vi "ECC.vi"() -> ()   [LabVIEW 2013]
uses:
  state_machine.ctl
  <vilib>/DAQmx/write.llb/DAQmx Write (Analog Wfm 1Chan NSamp).vi
  <vilib>/DAQmx/create/channels.llb/DAQmx Create Channel (AO-Voltage-Basic).vi
  <vilib>/DAQmx/configure/timing.llb/DAQmx Timing (Use Waveform).vi
  <vilib>/DAQmx/miscellaneous.llb/DAQmx Fill In Error Info.vi
panel:
  out "on_bad_status":bool
  out "off_bad_status":bool
  out "Pause, s":i32
  out "APS_off_status":bool=TRUE
  out "R&S_off_status":bool=TRUE
  out "Countdown":u32
  in  "Rep_delay":u32
  in  "Finite/Continuous":bool
  in  "ResumeSweep":bool
  in  "PauseSweep":bool
  in  "R&S_off_rep":bool
  in  "R&S_off_set":bool
  in  "R&S_off_cycle":bool
  in  "APS_off_rep":bool=TRUE
  in  "APS_off_set":bool
  in  "APS_off_cycle":bool
  in  "AbortSweep":bool
  in  "Check APS":bool
  in  "ON/OFF_APS":bool
  in  "Check R&S":bool
  in  "ON/OFF_R&S":bool
  in  "Use_APS":bool=TRUE
  out "DAC_status":bool
  out "R&S_status":bool
  out "i_Current_repetition":i32
  out "N_Cycles_Created":i32
  out "i_Current_cycle":i32
  in  "M_repetitions":i32 min=0
  in  "Set_of_Cycles":T1(array[cluster])=[{"On/Off"=TRUE, "f0, MHz"=32.5, "fm, kHz"=100.0, "A, mV"=20.0, "Waveform"=enum."triangle", "N_steps"=500, "T_sweep, s"=0.1, "N_sweeps"=5, "End_Wait, s"=0}] {"End_Wait, s" step=1; "N_sweeps" min=0 step=1; "T_sweep, s" min=0.0 step=0.001 format="%#_6f"; "N_steps" min=0 step=1; "fm, kHz" step=1.0; "f0, MHz" min=0.0 step=0.001 format="%#_6f"}
  out "APS_status":bool
  in  "APS address":refnum<visa-resource-name>="COM3"
  in  "Init Devices":bool
  in  "Do Sweep":bool
  in  "Exit":bool
  in  "DAC channel":tag="Dev1/ao0"
  in  "R&S address":string="29"
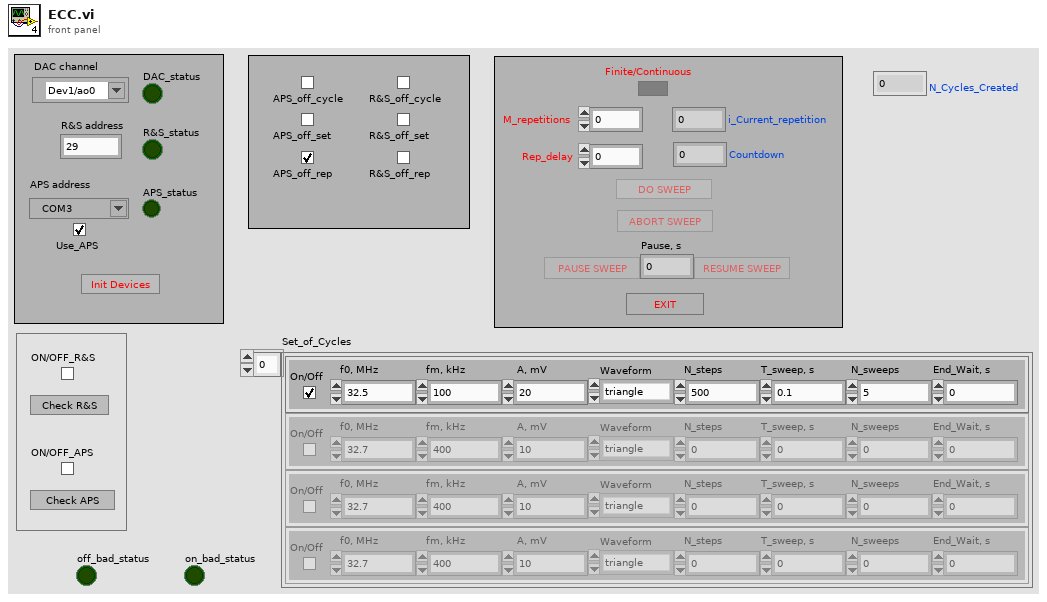
[diagram p1: front panel]
types:
  T1 = cluster{"On/Off":bool, "f0, MHz":dbl, "fm, kHz":dbl, "A, mV":dbl, "Waveform":enum16{"triangle", "saw_direct", "saw_invert", "sine"}, "N_steps":i32, "T_sweep, s":dbl, "N_sweeps":i32, "End_Wait, s":u32}[]
  T2 = typedef "state_machine.ctl" = enum16{"idle", "init_daq", "init_rf", "init_ps", "cycle_start", "get_wf", "rf_on", "rf_off", "rf_set", "ps_on", "ps_off", "daq_start", "daq_stop", "daq_wait", "daq_dt", "daq_v", "delay", "cycle_reset", "exit", "repetition_reset"}
  T3 = enum8{"Enabled", "Disabled", "Disabled and Grayed Out"}
  T4 = cluster{"On/Off":bool, "f0, MHz":dbl, "fm, kHz":dbl, "A, mV":dbl, "Waveform":enum16{"triangle", "saw_direct", "saw_invert", "sine"}, "N_steps":i32, "T_sweep, s":dbl, "N_sweeps":i32, "End_Wait, s":u32}
  T5 = enum16{"triangle", "saw_direct", "saw_invert", "sine"}
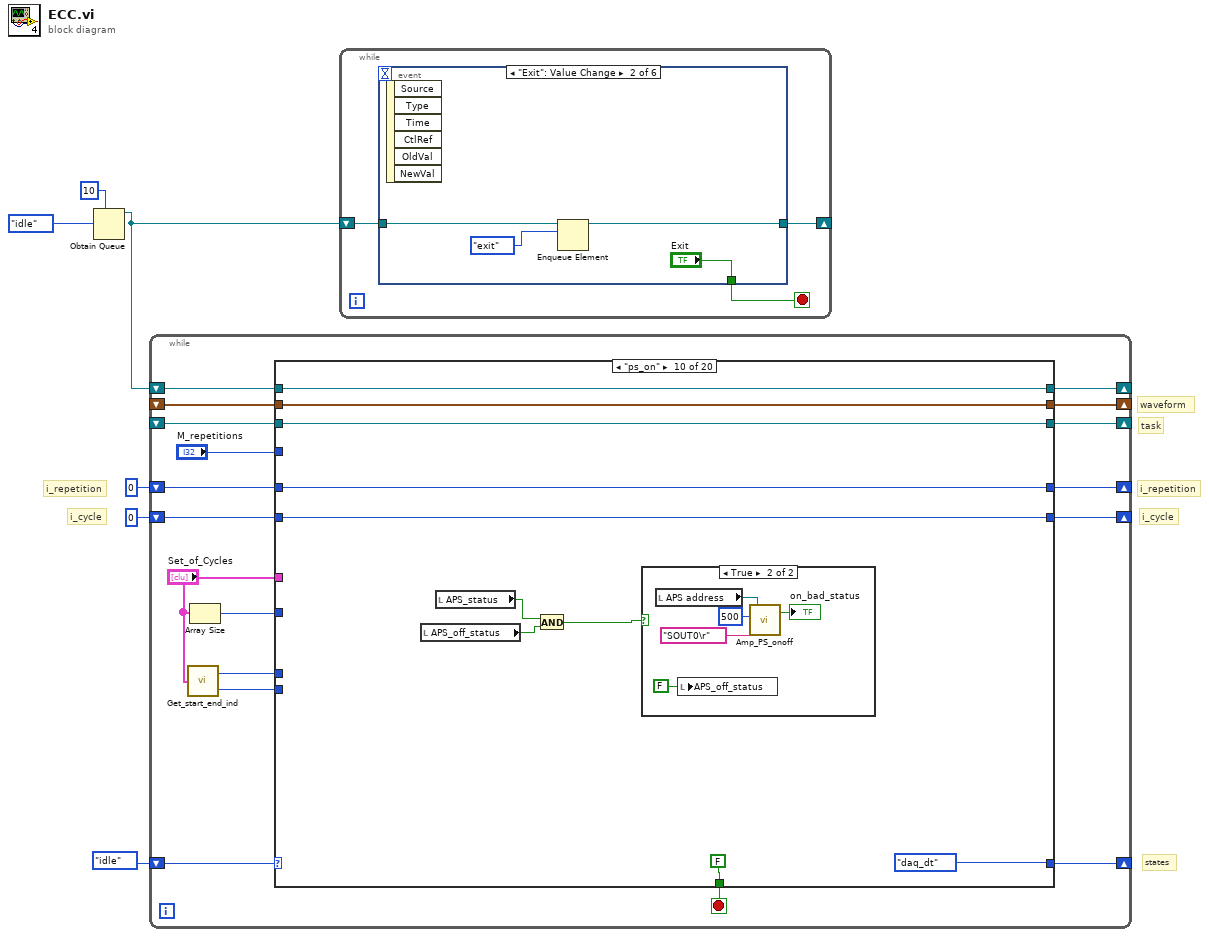
[diagram p0: block diagram]
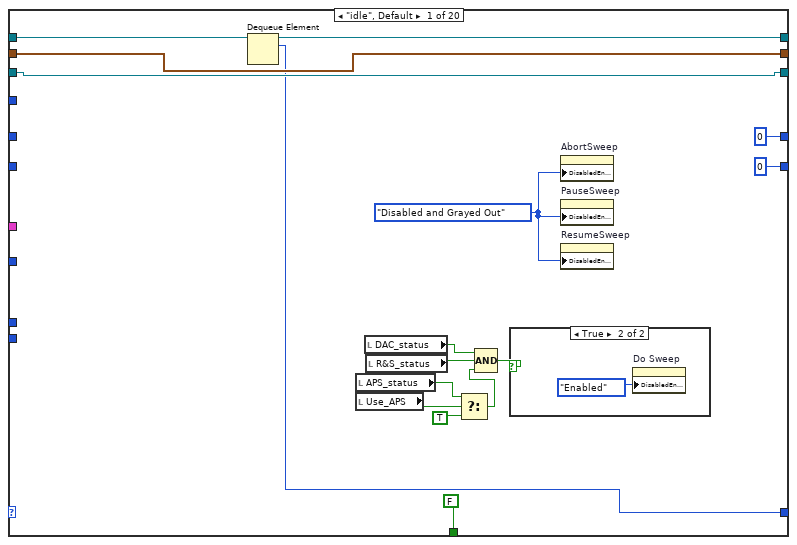
[diagram p2: hidden frame]
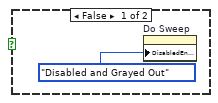
[diagram p3: hidden frame]
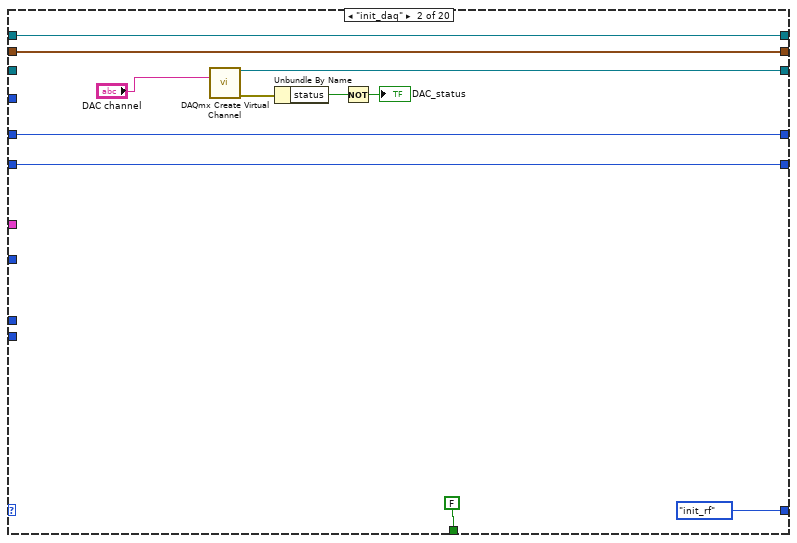
[diagram p4: hidden frame]
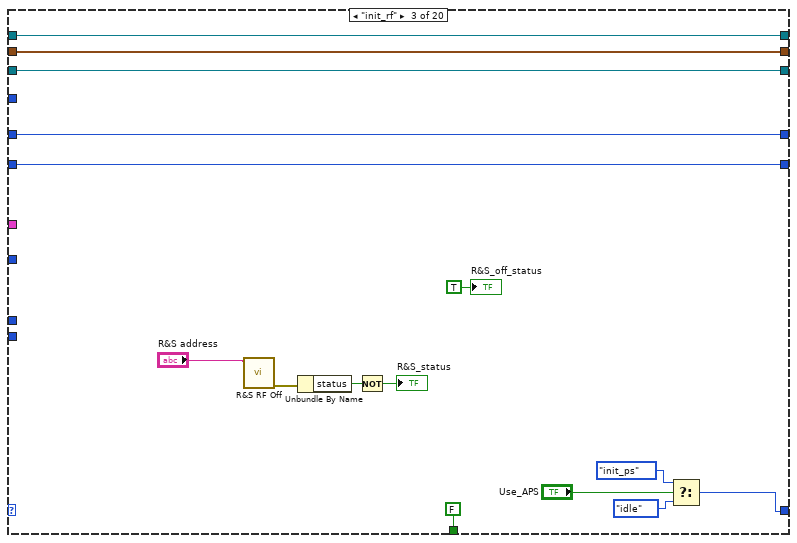
[diagram p5: hidden frame]
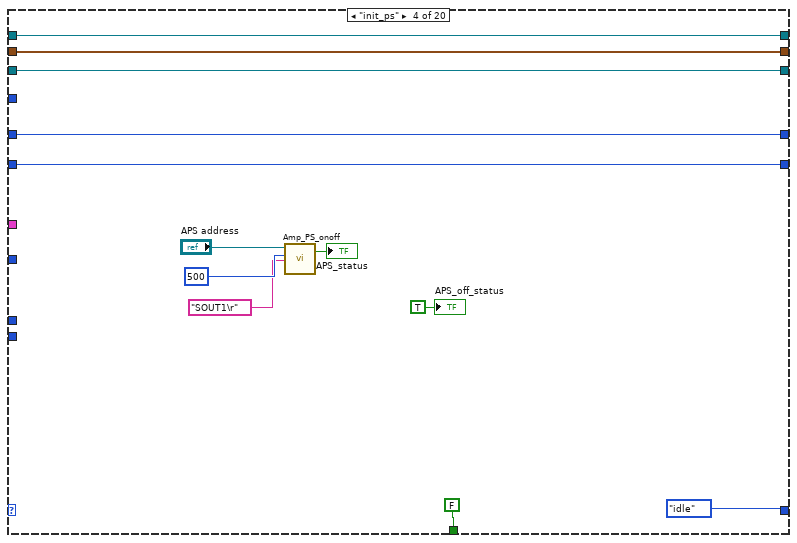
[diagram p6: hidden frame]
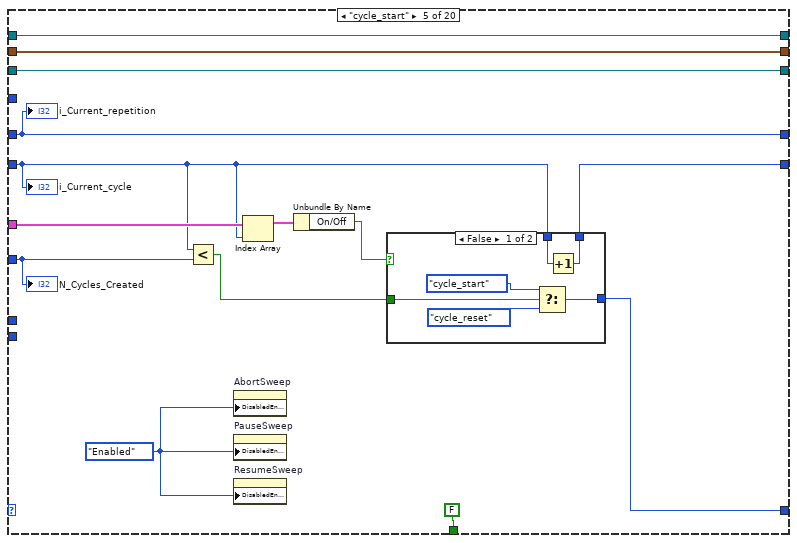
[diagram p7: hidden frame]
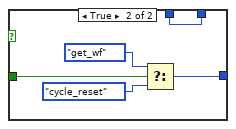
[diagram p8: hidden frame]
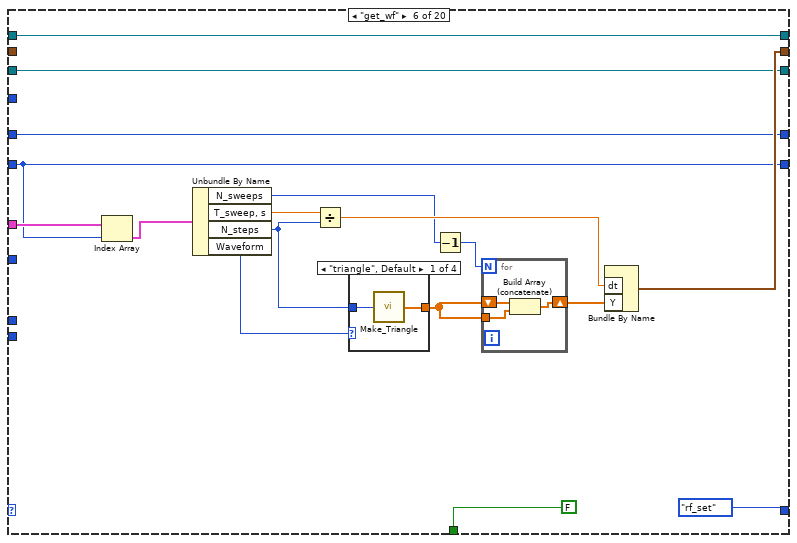
[diagram p9: hidden frame]
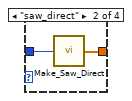
[diagram p10: hidden frame]
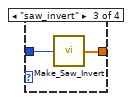
[diagram p11: hidden frame]
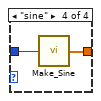
[diagram p12: hidden frame]
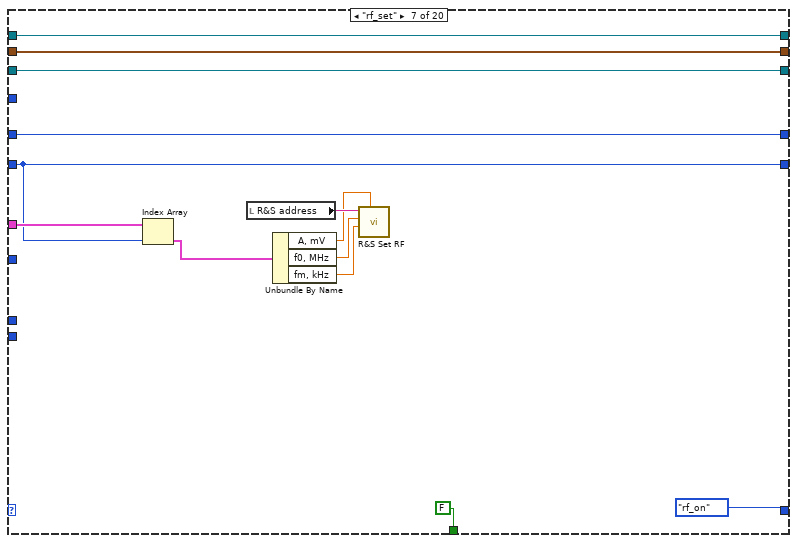
[diagram p13: hidden frame]
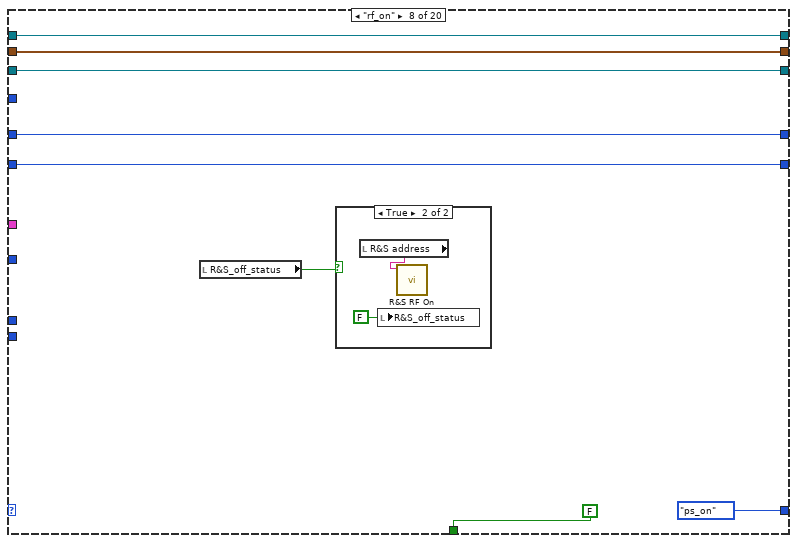
[diagram p14: hidden frame]
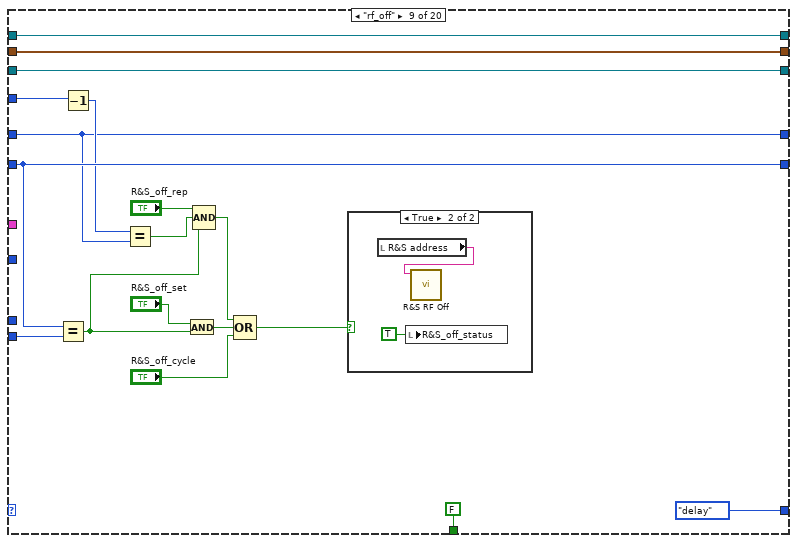
[diagram p16: hidden frame]
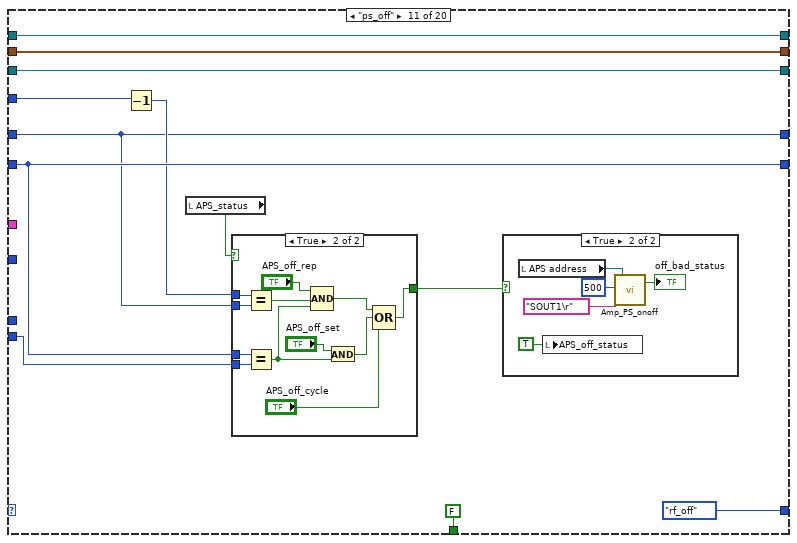
[diagram p19: hidden frame]
diagram:
  # "i_repetition"
  # "i_cycle"
  # "i_repetition"
  # "i_cycle"
  # "states"
  # "waveform"
  # "task"
  n1 = Obtain Queue(max queue size (-1, unlimited)=10, element data type=state_machine."idle") -> (queue out=w4:refnum<queue>)  [unwired: 3 in, 2 out]
  n2 = while {
    shift-right: [w19] -> _
    shift-left: state_machine."idle" -> [w24]
    shift-right: [w23] -> _
    shift-left: _ -> [w21]
    shift-right: [w22] -> _
    shift-left: _ -> [w20]
    shift-right: [w17] -> _
    shift-left: w4 -> [w18]
    shift-right: [w15] -> _
    shift-left: 0 -> [w14]
    shift-right: [w13] -> _
    shift-left: 0 -> [w12]
    stop <- w16 stop-if-true
    n3 = call "Get_start_end_ind.vi"("Set_of_Cycles"="Set_of_Cycles") -> ("start_ind"=w9:i32, "end_ind"=w8:i32)
    n4 = Array Size(array="Set_of_Cycles") -> (size(s)=w11:i32)
    n5 = case shown="\"ps_on\"" w24 {
      selector: w24 -> [_ _ _ _ _ _ _ _ _ _ _ _ _ _ _ _ _ _ w340 _]
      tunnel: [w40 w52 w68 w80 w84 w115 w143 w152 w172 w186 w203 w228 w236 w244 w253 w260 w272 w290 w337 w348] -> w23
      tunnel: "Set_of_Cycles" -> [_ _ _ _ w94 w122 w145 _ _ _ _ _ _ _ _ _ w269 _ _ _]
      tunnel: [w39 w51 w67 w79 w85 w116 w142 w153 w173 w185 w202 w227 w235 w243 w252 w261 w273 w289 w336 w349] -> w22
      tunnel: w21 -> [w40 _ w68 w80 w84 w115 w143 w152 w172 w186 w203 w229 w237 w245 w254 w262 w272 w290 w337 w348]
      tunnel: w20 -> [w39 w51 w67 w79 w85 _ w142 w153 w173 w185 w202 w227 w235 w243 w252 w261 w273 w289 w336 w349]
      tunnel: [w36 state_machine."init_rf" w58 state_machine."idle" w90 state_machine."rf_set" state_machine."rf_on" state_machine."ps_on" state_machine."delay" state_machine."daq_dt" state_machine."rf_off" state_machine."daq_wait" state_machine."ps_off" state_machine."daq_stop" state_machine."daq_v" state_machine."daq_start" state_machine."cycle_start" w288 w340 w344] -> w19
      tunnel: w18 -> [w38 w48 w65 w76 w83 w113 w140 w154 w174 w182 w199 w224 w232 w240 w248 w257 w274 w291 w339 w351]
      tunnel: [w37 w48 w65 w76 w83 w113 w140 w154 w174 w182 w199 w224 w232 w240 w248 w257 w274 w291 w339 w351] -> w17
      tunnel: [FALSE FALSE FALSE FALSE FALSE FALSE FALSE FALSE FALSE FALSE FALSE FALSE FALSE FALSE FALSE FALSE FALSE FALSE TRUE FALSE] -> w16
      tunnel: w11 -> [_ _ _ _ w86 _ _ _ _ _ _ _ _ _ _ _ _ _ _ _]
      tunnel: [0 w47 w64 w75 w89 w106 w138 w148 w168 w180 w197 w223 w231 w239 w247 w256 w264 0 w335 w350] -> w15
      tunnel: w14 -> [_ w47 w64 w75 w87 w106 w138 w148 w168 w180 w197 w223 w231 w239 w247 w256 w263 _ w335 w350]
      tunnel: [0 w46 w63 w74 w82 w108 w139 w151 w160 w181 w192 w222 w230 w238 w246 w255 w271 w285 w334 0] -> w13
      tunnel: w12 -> [_ w46 w63 w74 w82 w108 w139 w151 w160 w181 w192 w222 w230 w238 w246 w255 w271 w286 w334 _]
      tunnel: "M_repetitions" -> [_ _ _ _ _ _ _ _ w165 _ w194 _ _ _ _ _ _ w293 _ _]
      tunnel: w9 -> [_ _ _ _ _ _ _ _ _ _ _ _ _ _ _ _ _ _ _ _]
      tunnel: w8 -> [_ _ _ _ _ _ _ _ w169 _ w198 _ _ _ _ _ _ _ _ _]
      frame "idle", Default {
        w25 = T3."Disabled and Grayed Out" ("Disabled")
        n6 = Dequeue Element(queue=w38) -> (queue out=w37:refnum<queue>, element=w36:T2)  [unwired: 2 in, 2 out]
        n7 = local read "APS_status"() -> (w28:bool)
        n8 = local read "Use_APS"() -> (w30:bool)
        n9 = local read "DAC_status"() -> (w32:bool)
        n10 = local read "R&S_status"() -> (w31:bool)
        n11 = Select(t=w28, s=w30, f=TRUE) -> (s? t:f=w27:bool)
        n12 = Compound Arithmetic op=AND(w32, w31, w27) -> (w26:bool)
        n13 = case shown="True" w26 {
          frame False {
            n14 = property on="Do Sweep" class="Bool"("DisabledEnum"=T3."Disabled and Grayed Out" ("Disabled")) -> ()  [unwired: 2 in, 2 out]
          }
          frame True {
            n15 = property on="Do Sweep" class="Bool"("DisabledEnum"=T3."Enabled" ("Disabled")) -> ()  [unwired: 2 in, 2 out]
          }
        }
        n16 = property on="AbortSweep" class="Bool"("DisabledEnum"=w25) -> ()  [unwired: 2 in, 2 out]
        n17 = property on="PauseSweep" class="Bool"("DisabledEnum"=w25) -> ()  [unwired: 2 in, 2 out]
        n18 = property on="ResumeSweep" class="Bool"("DisabledEnum"=w25) -> ()  [unwired: 2 in, 2 out]
      }
      frame "init_daq" {
        n19 = call-poly <vilib>:"DAQmx Create Virtual Channel.vi"("physical channels"="DAC channel") -> ("task out"=w52:refnum<k21>, "error out"=w45:errorcluster)  [unwired: 13 in]
        n20 = Unbundle By Name(w45) -> ("status"=w44:bool)
        n21 = Not(x=w44) -> (.not. x?=→"DAC_status":bool)
      }
      frame "init_rf" {
        n22 = call "R&S RF Off.vi"("address"="R&S address") -> ("error out"=w54:errorcluster)  [unwired: 5 in, 1 out]
        n23 = Unbundle By Name(w54) -> ("status"=w61:bool)
        n24 = Not(x=w61) -> (.not. x?=→"R&S_status":bool)
        n25 = Select(t=state_machine."init_ps", s="Use_APS", f=state_machine."idle") -> (s? t:f=w58:T2)
        "R&S_off_status" <- TRUE ("R&S_off_status")
      }
      frame "init_ps" {
        n26 = call "Amp_PS_onoff.vi"("On/Off Control"="SOUT1\r", "delay before read (ms)"=u32 500, "Amp PS address"="APS address") -> ("status"=→"APS_status":bool)  [unwired: 1 in, 1 out]
        "APS_off_status" <- TRUE ("APS_off_status")
      }
      frame "cycle_start" {
        w81 = T3."Enabled" ("Disabled")
        n27 = Less?(x=w87, y=w86) -> (x < y?=w91:bool)
        n28 = property on="AbortSweep" class="Bool"("DisabledEnum"=w81) -> ()  [unwired: 2 in, 2 out]
        n29 = property on="PauseSweep" class="Bool"("DisabledEnum"=w81) -> ()  [unwired: 2 in, 2 out]
        n30 = property on="ResumeSweep" class="Bool"("DisabledEnum"=w81) -> ()  [unwired: 2 in, 2 out]
        n31 = Index Array(array=w94, index=w87) -> (element=w93:T4)
        n32 = Unbundle By Name(w93) -> ("On/Off"=w92:bool)
        n33 = case shown="False" w92 {
          tunnel: w91 -> [w98 w104]
          tunnel: [w95 w103] -> w90
          tunnel: w87 -> [w100 w101]
          tunnel: [w99 w101] -> w89
          frame False {
            n34 = Select(t=state_machine."cycle_start", s=w98, f=state_machine."cycle_reset") -> (s? t:f=w95:T2)
            n35 = Increment(x=w100) -> (x+1=w99:i32)
          }
          frame True {
            n36 = Select(t=state_machine."get_wf", s=w104, f=state_machine."cycle_reset") -> (s? t:f=w103:T2)
          }
        }
        "N_Cycles_Created" <- w86
        "i_Current_cycle" <- w87
        "i_Current_repetition" <- w82
      }
      frame "get_wf" {
        n37 = Index Array(array=w122, index=w106) -> (element=w121:T4)
        n38 = Unbundle By Name(w121) -> ("N_sweeps"=w112:i32, "T_sweep, s"=w110:dbl, "N_steps"=w109:i32, "Waveform"=w111:T5)
        n39 = Divide(x=w110, y=w109) -> (x/y=w118:dbl)
        n40 = case shown="\"triangle\", Default" w111 {
          tunnel: w109 -> [w127 w129 w131 w133]
          tunnel: [w126 w128 w130 w132] -> w119
          frame "triangle", Default {
            n41 = call "Make_Triangle.vi"("N_steps_1"=w127) -> ("TriangleWaveform"=w126:dbl[])
          }
          frame "saw_direct" {
            n42 = call "Make_Saw_Direct.vi"("N_steps_1"=w129) -> ("SawDirectWaveform"=w128:dbl[])
          }
          frame "saw_invert" {
            n43 = call "Make_Saw_Invert.vi"("N_steps_1"=w131) -> ("SawInvertWaveform"=w130:dbl[])
          }
          frame "sine" {
            n44 = call "Make_Sine.vi"("N_steps_1"=w133) -> ("SineWaveform"=w132:dbl[])
          }
        }
        n45 = Decrement(x=w112) -> (x-1=w117:i32)
        n46 = for {
          N: w117 -> [_]
          shift-right: [w123] -> w120
          shift-left: w119 -> [w125]
          tunnel: w119 -> [w124]
          n47 = Build Array (concatenate)(w125, w124) -> (w123:dbl[])
        }
        n48 = Bundle By Name("dt"=w118, "Y"=w120) -> (w116:waveform(dbl))  [unwired: 1 in]
      }
      frame "rf_set" {
        n49 = Index Array(array=w145, index=w138) -> (element=w144:T4)
        n50 = local read "R&S address"() -> (w146:string)
        n51 = Unbundle By Name(w144) -> ("A, mV"=w137:dbl, "f0, MHz"=w136:dbl, "fm, kHz"=w135:dbl)
        n52 = call "R&S Set RF.vi"("amplitude (mV)"=w137, "modulation (kHz)"=w135, "center frequency (MHz)"=w136, "address"=w146) -> ()  [unwired: 3 in, 2 out]
      }
      frame "rf_on" {
        n53 = local read "R&S_off_status"() -> (w147:bool)
        n54 = case shown="True" w147 {
          frame False {
          }
          frame True {
            n55 = local read "R&S address"() -> (w156:string)
            n56 = local write "R&S_off_status"(FALSE ("R&S_off_status")) -> ()
            n57 = call "R&S RF On.vi"("address"=w156) -> ()  [unwired: 5 in, 2 out]
          }
        }
      }
      frame "rf_off" {
        n58 = Equal?(x=w168, y=w169) -> (x = y?=w157:bool)
        n59 = Decrement(x=w165) -> (x-1=w161:i32)
        n60 = Equal?(x=w161, y=w160) -> (x = y?=w158:bool)
        n61 = And(x="R&S_off_set", y=w157) -> (x .and. y?=w164:bool)
        n62 = Compound Arithmetic op=AND("R&S_off_rep", w158, w157) -> (w162:bool)
        n63 = Compound Arithmetic op=OR(w162, w164, "R&S_off_cycle") -> (w166:bool)
        n64 = case shown="True" w166 {
          frame False {
          }
          frame True {
            n65 = local read "R&S address"() -> (w176:string)
            n66 = local write "R&S_off_status"(TRUE ("R&S_off_status")) -> ()
            n67 = call "R&S RF Off.vi"("address"=w176) -> ()  [unwired: 5 in, 2 out]
          }
        }
      }
      frame "ps_on" {
        n68 = local read "APS_off_status"() -> (w179:bool)
        n69 = local read "APS_status"() -> (w178:bool)
        n70 = And(x=w178, y=w179) -> (x .and. y?=w177:bool)
        n71 = case shown="True" w177 {
          frame False {
          }
          frame True {
            n72 = local read "APS address"() -> (w189:refnum<visa-resource-name>)
            n73 = local write "APS_off_status"(FALSE ("APS_off_status")) -> ()
            n74 = call "Amp_PS_onoff.vi"("On/Off Control"="SOUT0\r", "delay before read (ms)"=u32 500, "Amp PS address"=w189) -> ("status"=→"on_bad_status":bool)  [unwired: 1 in, 1 out]
          }
        }
      }
      frame "ps_off" {
        n75 = Decrement(x=w194) -> (x-1=w193:i32)
        n76 = local read "APS_status"() -> (w196:bool)
        n77 = case shown="True" w196 {
          selector: w196 -> [w204 _]
          tunnel: w198 -> [_ w216]
          tunnel: w197 -> [_ w215]
          tunnel: [w204 w210] -> w195
          tunnel: w193 -> [_ w206]
          tunnel: w192 -> [_ w207]
          frame False {
          }
          frame True {
            n78 = Equal?(x=w206, y=w207) -> (x = y?=w212:bool)
            n79 = Equal?(x=w215, y=w216) -> (x = y?=w205:bool)
            n80 = Compound Arithmetic op=AND("APS_off_rep", w212, w205) -> (w209:bool)
            n81 = And(x="APS_off_set", y=w205) -> (x .and. y?=w211:bool)
            n82 = Compound Arithmetic op=OR(w209, w211, "APS_off_cycle") -> (w210:bool)
          }
        }
        n83 = case shown="True" w195 {
          frame False {
          }
          frame True {
            n84 = local read "APS address"() -> (w219:refnum<visa-resource-name>)
            n85 = local write "APS_off_status"(TRUE ("APS_off_status")) -> ()
            n86 = call "Amp_PS_onoff.vi"("On/Off Control"="SOUT1\r", "delay before read (ms)"=u32 500, "Amp PS address"=w219) -> ("status"=→"off_bad_status":bool)  [unwired: 1 in, 1 out]
          }
        }
      }
      frame "daq_start" {
        n87 = call <vilib>:"DAQmx Start Task.vi"("task/channels in"=w229) -> ("task out"=w228:refnum<k21>)  [unwired: 13 in, 1 out]
      }
      frame "daq_stop" {
        n88 = call <vilib>:"DAQmx Stop Task.vi"("task/channels in"=w237) -> ("task out"=w236:refnum<k21>)  [unwired: 13 in, 1 out]
      }
      frame "daq_wait" {
        n89 = call <vilib>:"DAQmx Wait Until Done.vi"("task/channels in"=w245) -> ("task out"=w244:refnum<k21>)  [unwired: 13 in, 1 out]
      }
      frame "daq_dt" {
        w251 = 10178 items=["Finite Samples"=10178, "Continuous Samples"=10123, "Hardware Timed Single Point"=12522] ("sample mode")
        n90 = call-poly <vilib>:"DAQmx Timing.vi"("task/channels in"=w254, "sample mode"=w251, "waveform"=w252) -> ("task out"=w253:refnum<k21>)  [unwired: 11 in, 1 out]
      }
      frame "daq_v" {
        n91 = call-poly <vilib>:"DAQmx Write.vi"("task/channels in"=w262, "data"=w261) -> ("task out"=w260:refnum<k21>)  [unwired: 11 in, 2 out]
      }
      frame "delay" {
        # "iterate cycle"
        n92 = Increment(x=w263) -> (x+1=w264:i32)
        n93 = Index Array(array=w269, index=w263) -> (element=w270:T4)
        n94 = Unbundle By Name(w270) -> ("End_Wait, s"=w267:u32)
        n95 = Equal To 0?(x=w267) -> (x = 0?=w268:bool)
        n96 = case shown="True" w268 {
          tunnel: w267 -> [w275 _]
          frame False {
            n97 = Multiply(x=u32 1000 ("y"), y=w275) -> (x*y=w277:u32)
            n98 = Wait (ms)(milliseconds to wait=w277) -> ()  [unwired: 1 out]
          }
          frame True {
          }
        }
      }
      frame "cycle_reset" {
        # "iterate repetition"
        n99 = Increment(x=w286) -> (x+1=w281:i32)
        n100 = case shown="True" "PauseSweep" {
          tunnel: [FALSE ("ResumeSweep") w306] -> w282
          frame False {
          }
          frame True {
            n101 = Tick Count (ms)() -> (millisecond timer value=w307:u32)
            n102 = while {
              tunnel: w307 -> [w313]
              tunnel: ["ResumeSweep"] -> w306
              stop <- "ResumeSweep" stop-if-true
              n103 = Tick Count (ms)() -> (millisecond timer value=w314:u32)
              n104 = Subtract(x=w314, y=w313) -> (x-y=w312:u32)
              n105 = Divide(x=w312, y=u32 1000) -> (x/y=w310:dbl)
              n106 = To Long Integer(number=w310) -> (32bit integer=→"Pause, s":i32)
            }
          }
        }
        n107 = Less?(x=w281, y=w293) -> (x < y?=w287:bool)
        n108 = Or(x="AbortSweep", y="PauseSweep") -> (x .or. y?=w278:bool)
        n109 = case shown="True" "AbortSweep" {
          tunnel: [w323 state_machine."idle"] -> w288
          tunnel: w287 -> [w322 _]
          tunnel: w281 -> [w321 _]
          tunnel: [w321 0] -> w285
          frame False {
            n110 = Select(t=state_machine."cycle_start", s=w322, f=state_machine."repetition_reset") -> (s? t:f=w323:T2)
          }
          frame True {
            w327 = T3."Enabled" ("Disabled")
            n111 = property on="Check APS" class="Bool"("DisabledEnum"=w327) -> ()  [unwired: 2 in, 2 out]
            n112 = property on="Check R&S" class="Bool"("DisabledEnum"=w327) -> ()  [unwired: 2 in, 2 out]
          }
        }
        n113 = case shown="True" w278 {
          frame False {
          }
          frame True {
            n114 = local write "R&S_off_status"(TRUE ("R&S_off_status")) -> ()
            n115 = local read "R&S address"() -> (w316:string)
            n116 = call "R&S RF Off.vi"("address"=w316) -> ()  [unwired: 5 in, 2 out]
          }
        }
        n117 = local read "APS_status"() -> (w279:bool)
        n118 = case shown="True" w282 {
          frame False {
          }
          frame True {
            n119 = local read "R&S_off_status"() -> (w300:bool)
            n120 = case shown="False" w300 {
              frame False {
                n121 = local read "R&S address"() -> (w304:string)
                n122 = call "R&S RF On.vi"("address"=w304) -> ()  [unwired: 5 in, 2 out]
              }
              frame True {
              }
            }
            n123 = local write "Pause, s"(0 ("Pause, s")) -> ()
            n124 = local read "APS_off_status"() -> (w298:bool)
            n125 = local read "APS_status"() -> (w299:bool)
            n126 = Not(x=w298) -> (.not. x?=w297:bool)
            n127 = And(x=w299, y=w297) -> (x .and. y?=w296:bool)
            n128 = case shown="True" w296 {
              frame False {
              }
              frame True {
                n129 = local read "APS address"() -> (w301:refnum<visa-resource-name>)
                n130 = call "Amp_PS_onoff.vi"("On/Off Control"="SOUT0\r", "delay before read (ms)"=u32 50, "Amp PS address"=w301) -> ()  [unwired: 1 in, 2 out]
              }
            }
          }
        }
        n131 = And(x=w278, y=w279) -> (x .and. y?=w280:bool)
        n132 = case shown="True" w280 {
          frame False {
          }
          frame True {
            n133 = local read "APS address"() -> (w318:refnum<visa-resource-name>)
            n134 = local write "APS_off_status"(TRUE ("APS_off_status")) -> ()
            n135 = call "Amp_PS_onoff.vi"("On/Off Control"="SOUT1\r", "delay before read (ms)"=u32 500, "Amp PS address"=w318) -> ()  [unwired: 1 in, 2 out]
          }
        }
      }
      frame "exit" {
        w329 = FALSE ("DAC_status")
        n136 = local read "APS address"() -> (w332:refnum<visa-resource-name>)
        n137 = local read "Use_APS"() -> (w333:bool)
        n138 = local read "R&S address"() -> (w331:string)
        n139 = case shown="False" w333 {
          tunnel: w332 -> [_ w341]
          frame False {
          }
          frame True {
            n140 = call "Amp_PS_onoff.vi"("On/Off Control"="SOUT1\r", "delay before read (ms)"=u32 50, "Amp PS address"=w341) -> ()  [unwired: 1 in, 2 out]
          }
        }
        n141 = call "R&S RF Off.vi"("address"=w331) -> ()  [unwired: 5 in, 2 out]
        n142 = property on="Init Devices" class="Bool"("DisabledEnum"=T3."Enabled" ("Disabled")) -> ()  [unwired: 2 in, 2 out]
        n143 = local write "DAC_status"(w329) -> ()
        n144 = local write "R&S_status"(w329) -> ()
        n145 = local write "APS_status"(w329) -> ()
      }
      frame "repetition_reset" {
        n146 = case shown="True" "Finite/Continuous" {
          tunnel: [state_machine."idle" state_machine."cycle_start"] -> w344
          frame False {
          }
          frame True {
            n147 = Tick Count (ms)() -> (millisecond timer value=w354:u32)
            n148 = while {
              tunnel: w354 -> [w361]
              tunnel: "Rep_delay" -> [w357]
              stop <- w359 stop-if-true
              w356 = u32 1000 ("y")
              n149 = Tick Count (ms)() -> (millisecond timer value=w362:u32)
              n150 = Subtract(x=w362, y=w361) -> (x-y=w363:u32)
              n151 = Divide(x=w363, y=w356) -> (x/y=w364:dbl)
              n152 = Wait (ms)(milliseconds to wait=w356) -> ()  [unwired: 1 out]
              n153 = To Long Integer(number=w364) -> (32bit integer=w358:i32)
              n154 = Subtract(x=w357, y=w358) -> (x-y=w360:u32)
              "Countdown" <- w360
              n155 = Less Or Equal To 0?(x=w360) -> (x <= 0?=w359:bool)
            }
          }
        }
      }
    }
  }
  n156 = while {
    shift-right: [w365] -> _
    shift-left: w4 -> [w366]
    stop <- w367 stop-if-true
    n157 = event shown="[1] \"Exit\": Value Change" {
      selector: _ -> [_ _ _ _ _ _]
      dyn-events: _ -> [_ _ _ _ _ _]
      timeout: _ -> [_ _ _ _ _ _]
      tunnel: [_ "Exit" w377 w383 w389 w396] -> w367
      tunnel: w366 -> [w368 w371 w376 w382 w386 w393]
      tunnel: [w368 w370 w375 w381 w386 w393] -> w365
      event Timeout {
        n158 = event-data() -> ()  [unwired: 1 in, 3 out]
      }
      event "Exit": Value Change {
        n159 = event-data() -> ()  [unwired: 1 in, 6 out]
        n160 = Enqueue Element(queue=w371, element=state_machine."exit") -> (queue out=w370:refnum<queue>)  [unwired: 2 in, 2 out]
      }
      event "Init Devices": Value Change {
        n161 = event-data() -> ()  [unwired: 1 in, 6 out]
        n162 = Enqueue Element(queue=w376, element=state_machine."init_daq") -> (queue out=w375:refnum<queue>)  [unwired: 2 in, 2 out]
        n163 = property on="Init Devices" class="Bool"("DisabledEnum"=T3."Disabled and Grayed Out" ("Disabled")) -> ()  [unwired: 2 in, 2 out]
        n164 = Not(x="Init Devices") -> (.not. x?=w377:bool)
      }
      event "Do Sweep": Value Change {
        w379 = T3."Disabled and Grayed Out" ("Disabled")
        n165 = event-data() -> ()  [unwired: 1 in, 6 out]
        n166 = Enqueue Element(queue=w382, element=state_machine."cycle_start") -> (queue out=w381:refnum<queue>)  [unwired: 2 in, 2 out]
        n167 = Not(x="Do Sweep") -> (.not. x?=w383:bool)
        n168 = property on="Check R&S" class="Bool"("DisabledEnum"=w379) -> ()  [unwired: 2 in, 2 out]
        n169 = property on="Check APS" class="Bool"("DisabledEnum"=w379) -> ()  [unwired: 2 in, 2 out]
      }
      event "Check R&S": Value Change {
        n170 = event-data() -> ()  [unwired: 1 in, 6 out]
        n171 = local read "R&S address"() -> (w387:string)
        n172 = case shown="True" "ON/OFF_R&S" {
          tunnel: w387 -> [w390 w391]
          frame False {
            n173 = call "R&S RF Off.vi"("address"=w390) -> ()  [unwired: 5 in, 2 out]
          }
          frame True {
            n174 = call "R&S RF On.vi"("address"=w391) -> ()  [unwired: 5 in, 2 out]
          }
        }
        n175 = Not(x="Check R&S") -> (.not. x?=w389:bool)
      }
      event "Check APS": Value Change {
        n176 = event-data() -> ()  [unwired: 1 in, 6 out]
        n177 = local read "APS address"() -> (w394:refnum<visa-resource-name>)
        n178 = case shown="False" "ON/OFF_APS" {
          tunnel: w394 -> [w397 w400]
          frame False {
            n179 = call "Amp_PS_onoff.vi"("On/Off Control"="SOUT1\r", "delay before read (ms)"=u32 50, "Amp PS address"=w397) -> ()  [unwired: 1 in, 2 out]
          }
          frame True {
            n180 = call "Amp_PS_onoff.vi"("On/Off Control"="SOUT0\r", "delay before read (ms)"=u32 50, "Amp PS address"=w400) -> ()  [unwired: 1 in, 2 out]
          }
        }
        n181 = Not(x="Check APS") -> (.not. x?=w396:bool)
      }
    }
  }
